vi "PRL UTIL Split Command.vi"(11 "Command":string) -> (2 "Parameters":string, 3 "Command Out":string)   [LabVIEW 2018, in "S3DK.lvlib" / "PMU Recorder Light.lvlib"]
doc: "Splits the command string into command and sub-command."
uses:
  .S3DK - Copy/PMU Recorder Light/PMU Recorder Light.lvlib
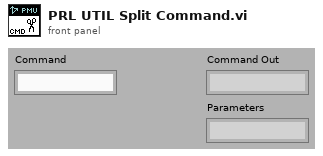
[diagram p1: front panel]
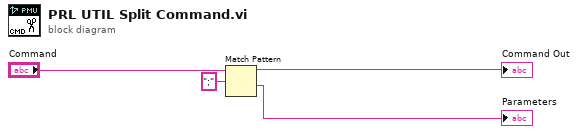
[diagram p0: block diagram]
diagram:
  n1 = Match Pattern(string="Command", regular expression=";") -> (before substring=→"Command Out":string, after substring=→"Parameters":string)  [unwired: 1 in, 2 out]
